vi "Ke2000 Reading MilAmp_jose.vi"(0 "VISA resource name":refnum<visa-resource-name>, 11 "error in (no error)":errorcluster) -> (4 "VISA resource name out":refnum<visa-resource-name>, 6 "uA":string, 10 "error out":errorcluster, 15 "Mili Amp":dbl)   [LabVIEW 2009]
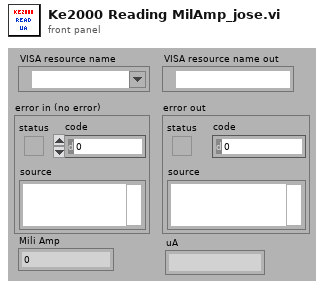
[diagram p1: front panel]
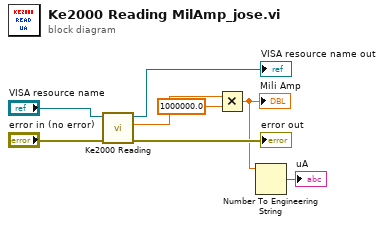
[diagram p0: block diagram]
diagram:
  n1 = call "Ke2000 Reading.vi"("error in (no error)"="error in (no error)", "VISA resource name"="VISA resource name") -> ("error out"=→"error out":errorcluster, "Measurement"=w6:dbl, "VISA resource name out"=→"VISA resource name out":refnum<visa-resource-name>)  [unwired: 6 in, 1 out]
  n2 = Multiply(x=w6, y=1000000.0) -> (x*y=w2:dbl)
  "Mili Amp" <- w2
  n3 = Number To Engineering String(4:w2) -> (0:→"uA":string)  [unwired: 3 in]
